vi "laserDiagnose_UV.vi"(0 "320 Port":refnum<visa-resource-name>, 5 "375 Port in":refnum<visa-resource-name>, 7 "445 Port 3":refnum<visa-resource-name>, 11 "error in (no error)":errorcluster, 12 "ms to wait (50)":u32=50) -> (4 "Powers":T3, 6 "Currents":T1, 8 "Temperatures":T2, 10 "Overtemp":bool, 15 "error out":errorcluster)   [LabVIEW 2011]
panel:
  out "445 Port Out":refnum<visa-resource-name>
  out "375 Port Out":refnum<visa-resource-name>
  out "320 Port Out":refnum<visa-resource-name>
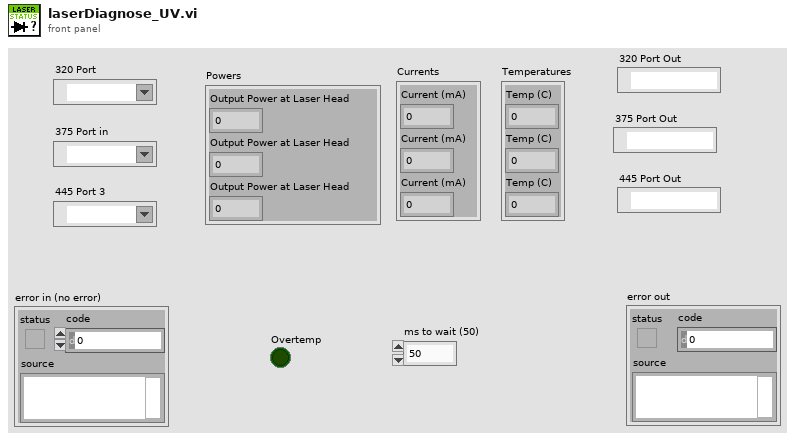
[diagram p1: front panel]
types:
  T1 = cluster{"Current (mA)":dbl, "Current (mA)":dbl, "Current (mA)":dbl}
  T2 = cluster{"Temp (C)":dbl, "Temp (C)":dbl, "Temp (C)":dbl}
  T3 = cluster{"Output Power at Laser Head":dbl, "Output Power at Laser Head":dbl, "Output Power at Laser Head":dbl}
  T4 = cluster{"Laser Diode Temp (C)":dbl, "Temp (C)":dbl, "Temp (C)":dbl}
  T5 = cluster{"Laser Diode Current":dbl, "Current, mA":dbl, "Current, mA":dbl}
  T6 = cluster{"Laser Diode Power":dbl, "Power, mW":dbl, "Power, mW":dbl}
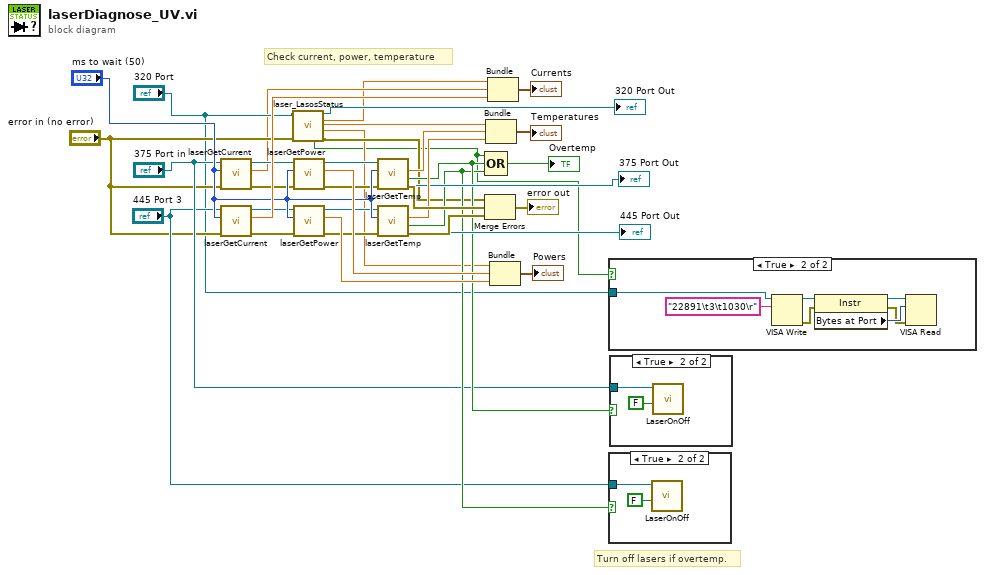
[diagram p0: block diagram]
diagram:
  # "Check current, power, temperature"
  # "Turn off lasers if overtemp."
  n1 = call "laserGetCurrent.vi"("error in (no error)"="error in (no error)", "ms to wait (5)"="ms to wait (50)", "VISA resource name"="375 Port in") -> ("error out"=w22:errorcluster, "Current, mA"=w7:dbl, "VISA resource name out"=w18:refnum<visa-resource-name>)  [unwired: 6 in]
  n2 = call "laserGetCurrent.vi"("error in (no error)"="error in (no error)", "ms to wait (5)"="ms to wait (50)", "VISA resource name"="445 Port 3") -> ("error out"=w25:errorcluster, "Current, mA"=w27:dbl, "VISA resource name out"=w20:refnum<visa-resource-name>)  [unwired: 6 in]
  n3 = call "laser_LasosStatus.vi"("VISA Refnum in"="320 Port", "error in (no error)"="error in (no error)") -> ("VISA Refnum out"=→"320 Port Out":refnum<visa-resource-name>, "Laser Diode Current"=w4:dbl, "Laser Diode Temp (C)"=w5:dbl, "Laser Diode Power"=w3:dbl, "Overtemp?"=w1:bool, "error out"=w8:errorcluster)  [unwired: 8 in]
  n4 = call "laserGetPower.vi"("error in (no error)"=w22, "ms to wait (5)"="ms to wait (50)", "VISA resource name"=w18) -> ("error out"=w23:errorcluster, "Power, mW"=w31:dbl, "VISA resource name out"=w19:refnum<visa-resource-name>)  [unwired: 6 in]
  n5 = call "laserGetPower.vi"("error in (no error)"=w25, "ms to wait (5)"="ms to wait (50)", "VISA resource name"=w20) -> ("error out"=w24:errorcluster, "Power, mW"=w32:dbl, "VISA resource name out"=w21:refnum<visa-resource-name>)  [unwired: 6 in]
  n6 = call "laserGetTemp.vi"("error in (no error)"=w23, "milliseconds to wait"="ms to wait (50)", "VISA resource name"=w19) -> ("error out"=w34:errorcluster, "Overtemp"=w14:bool, "Temp (C)"=w29:dbl, "VISA resource name out"=→"375 Port Out":refnum<visa-resource-name>)  [unwired: 5 in]
  n7 = call "laserGetTemp.vi"("error in (no error)"=w24, "milliseconds to wait"="ms to wait (50)", "VISA resource name"=w21) -> ("error out"=w35:errorcluster, "Overtemp"=w13:bool, "Temp (C)"=w30:dbl, "VISA resource name out"=→"445 Port Out":refnum<visa-resource-name>)  [unwired: 5 in]
  n8 = Compound Arithmetic op=OR(w1, w14, w13) -> (→"Overtemp":bool)
  n9 = Merge Errors(w8, w34, w35) -> (→"error out":errorcluster)
  n10 = Bundle("Laser Diode Temp (C)"=w5, "Temp (C)"=w29, "Temp (C)"=w30) -> (→"Temperatures":T4)  [unwired: 1 in]
  n11 = Bundle("Laser Diode Current"=w4, "Current, mA"=w7, "Current, mA"=w27) -> (→"Currents":T5)  [unwired: 1 in]
  n12 = Bundle("Laser Diode Power"=w3, "Power, mW"=w31, "Power, mW"=w32) -> (→"Powers":T6)  [unwired: 1 in]
  n13 = case shown="True" w1 {
    tunnel: "320 Port" -> [_ w37]
    frame False {
    }
    frame True {
      n14 = VISA Write(VISA resource name=w37, write buffer="22891\t3\t1030\r") -> (VISA resource name out=w38:refnum<visa-resource-name>, error out=w39:errorcluster)  [unwired: 1 in, 1 out]
      n15 = property class="Instr"(reference=w38, error in=w39) -> (reference out=w40:refnum<visa-resource-name>, error out=w41:errorcluster, "Bytes at Port"=w42:u32)
      n16 = VISA Read(VISA resource name=w40, byte count=w42, error in (no error)=w41) -> ()  [unwired: 4 out]
    }
  }
  n17 = case shown="True" w13 {
    tunnel: "445 Port 3" -> [_ w45]
    frame False {
    }
    frame True {
      n18 = call "LaserOnOff.vi"("Emission (F = OFF)"=FALSE ("405 Emission (T = ON)"), "VISA Refnum in"=w45) -> ()  [unwired: 7 in, 3 out]
    }
  }
  n19 = case shown="True" w14 {
    tunnel: "375 Port in" -> [_ w47]
    frame False {
    }
    frame True {
      n20 = call "LaserOnOff.vi"("Emission (F = OFF)"=FALSE ("405 Emission (T = ON)"), "VISA Refnum in"=w47) -> ()  [unwired: 7 in, 3 out]
    }
  }
